vi "close_refs.vi"(11 "Test Data in":T1) -> ()   [LabVIEW 2024, in "IPE Optimization Tester.lvlib"]
uses:
  IPE Optimization Tester.lvlib
  Tests/test_data--cluster.ctl
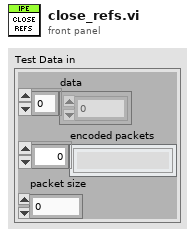
[diagram p1: front panel]
types:
  T1 = typedef "IPE Optimization Tester.lvlib/test_data--cluster.ctl" = cluster{"data":dbl[], "encoded packets":string[], "packet size":i32}
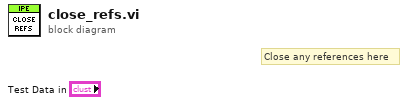
[diagram p0: block diagram]
diagram:
  # "Close any references here"
